vi "SerialWriteRead.vi"(8 "error in (no error)":errorcluster, 9 "Bytes to read":u32, 10 "The byte to send before reading":string caption="Opcode", 11 "VISA Refnum in":refnum<visa-resource-name>) -> (0 "error out":errorcluster, 1 "Hex Out":string, 2 "Error? Out":bool, 3 "VISA Refnum out":refnum<visa-resource-name>)   [LabVIEW 2013]
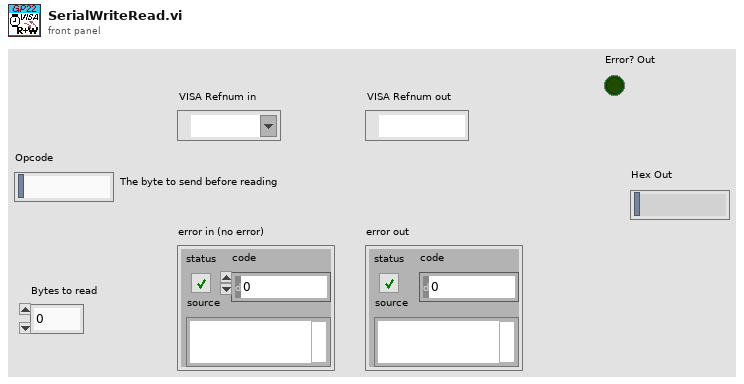
[diagram p1: front panel]
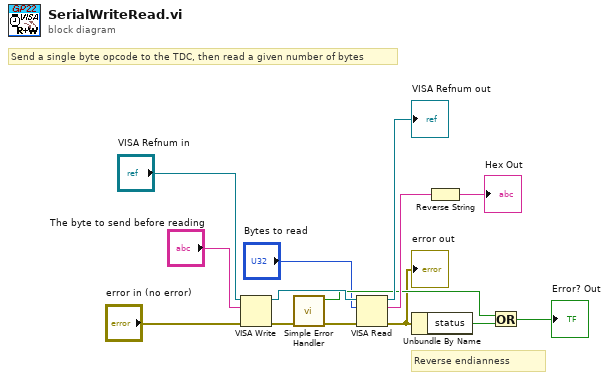
[diagram p0: block diagram]
diagram:
  # "Send a single byte opcode to the TDC, then read a given number of bytes"
  # "Reverse endianness"
  n1 = VISA Write(VISA resource name="VISA Refnum in", write buffer="The byte to send before reading", error in (no error)="error in (no error)") -> (VISA resource name out=w11:refnum<visa-resource-name>, error out=w10:errorcluster)  [unwired: 1 out]
  n2 = call <vilib>:"Simple Error Handler.vi"("error in (no error)"=w10) -> ("error?"=w5:bool, "error out"=w9:errorcluster)  [unwired: 4 in, 3 out]
  n3 = VISA Read(VISA resource name=w11, byte count="Bytes to read", error in (no error)=w9) -> (VISA resource name out=→"VISA Refnum out":refnum<visa-resource-name>, read buffer=w6:string, error out=w1:errorcluster)  [unwired: 1 out]
  "error out" <- w1
  n4 = Unbundle By Name(w1) -> ("status"=w2:bool)
  n5 = Reverse String(1:w6) -> (0:→"Hex Out":string)
  n6 = Or(x=w5, y=w2) -> (x .or. y?=→"Error? Out":bool)
